vi "IR-sensor_labview_finalVersion.vi"() -> ()   [LabVIEW 2018]
uses:
  Downloads/Communicatie-met-Arduino-met-StateMachine-met-EventStructure (1).ctl
  <vilib>/Instr/_visa.llb/VISA Configure Serial Port (Instr).vi
panel:
  in  "VISA resource name":refnum<visa-resource-name>
  out "Absorberen":dbl(slide) scale=0.0..500.0
  in  "Clear Chart":bool
  out "Reflecteren":dbl(slide) scale=0.0..500.0
  out "Omgevings straling\nReferentie waarde":string
  in  "Kalibreren":bool
  out "Reflecteren":bool
  out "Absorberen":bool
  in  "Path":path
  out "Array":dbl[](array[numeric])
  in  "Wegschrijven":bool
  out "Status":T1
  in  "Baud rate":u32
  in  "Configure":bool
  in  "Stop":bool
  out "Waveform Chart":cluster{"decimal":u32, "Referentie":dbl}(graph)
  out "Huidige waarde":string
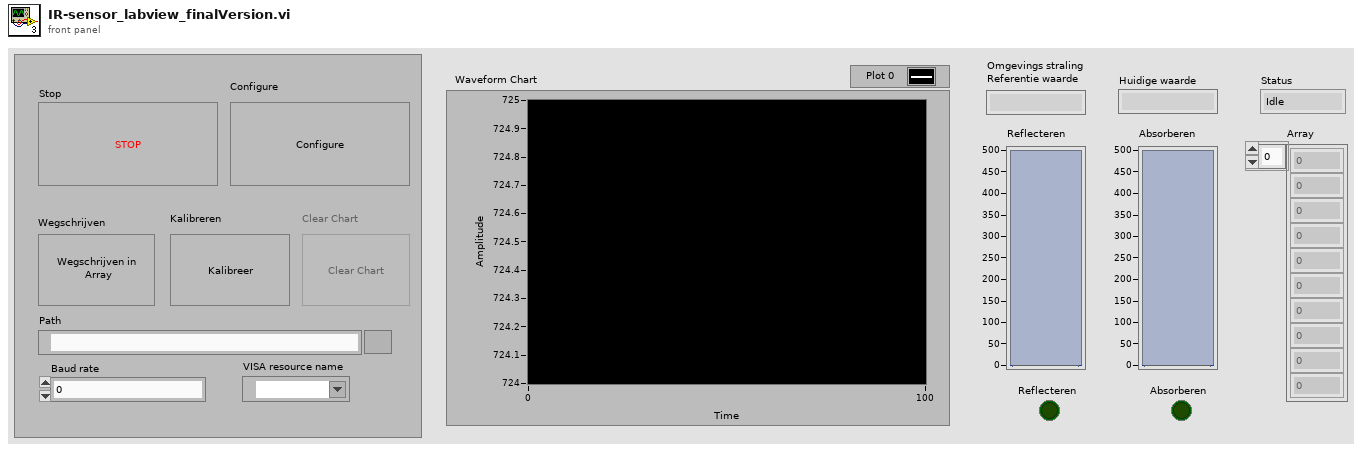
[diagram p1: front panel]
types:
  T1 = typedef "Communicatie-met-Arduino-met-StateMachine-met-EventStructure (1).ctl" = enum16{"Idle", "End", "Visualize", "Process", "Read", "Connect"}
  T2 = cluster{"COM Arduino":refnum<visa-resource-name>, "Baud rate 2":u32, "connect char":string, "buffer":string, "converted voltage":dbl, "decimal":u32, "value":i32, "saved values":dbl[], "refnum out":refnum<file>, "image":path, "ToArduino text":string, "Referentie":dbl}
  T3 = enum8{"Enabled", "Disabled", "Disabled and Grayed Out"}
  T4 = typedef "imagedata.ctl" = cluster{"image type":i32, "image depth":i32, "image":u8[], "mask":u8[], "colors":u32[], "Rectangle":cluster{"left":i16, "top":i16, "right":i16, "bottom":i16}}
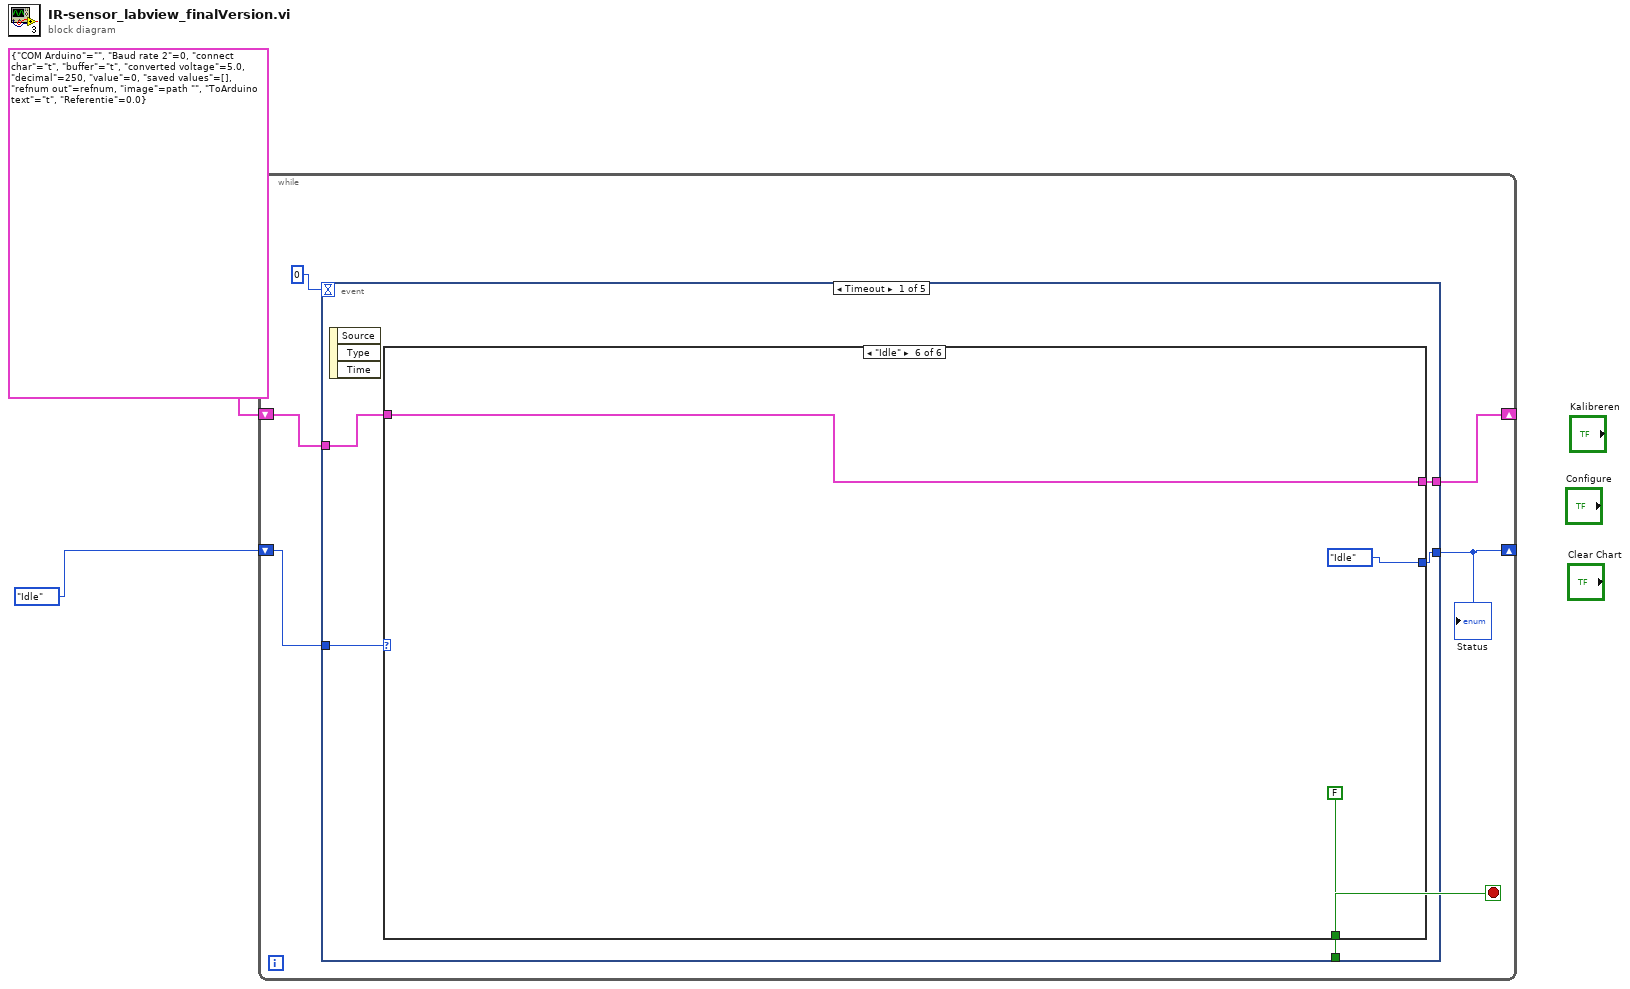
[diagram p0: block diagram]
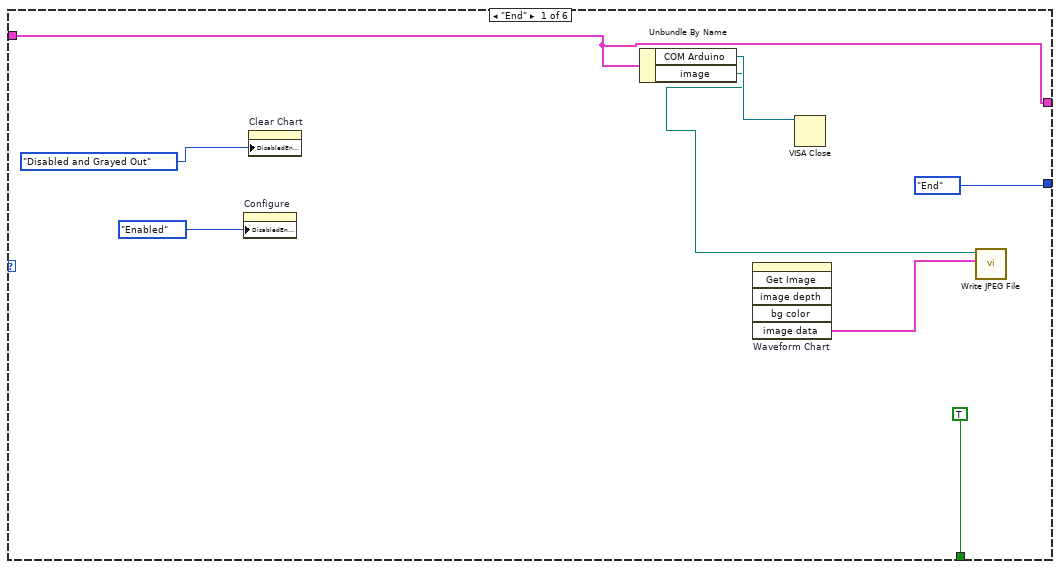
[diagram p2: hidden frame]
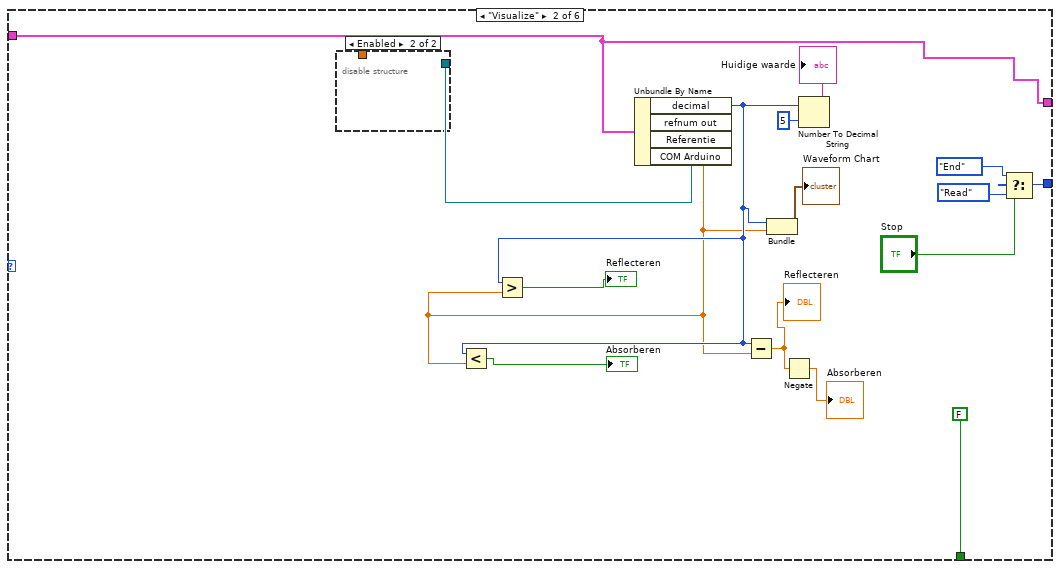
[diagram p3: hidden frame]
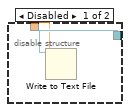
[diagram p4: hidden frame]
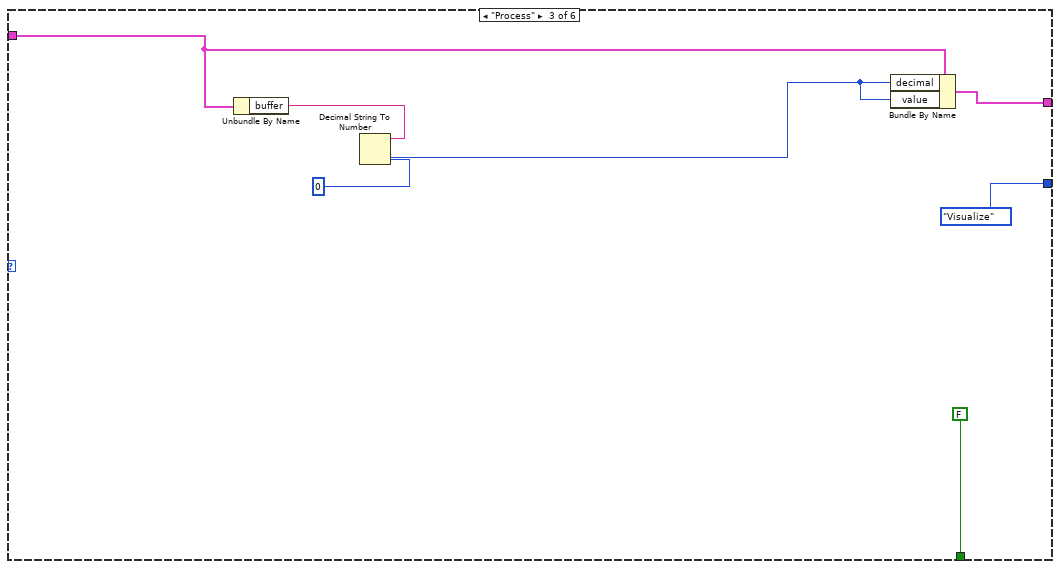
[diagram p5: hidden frame]
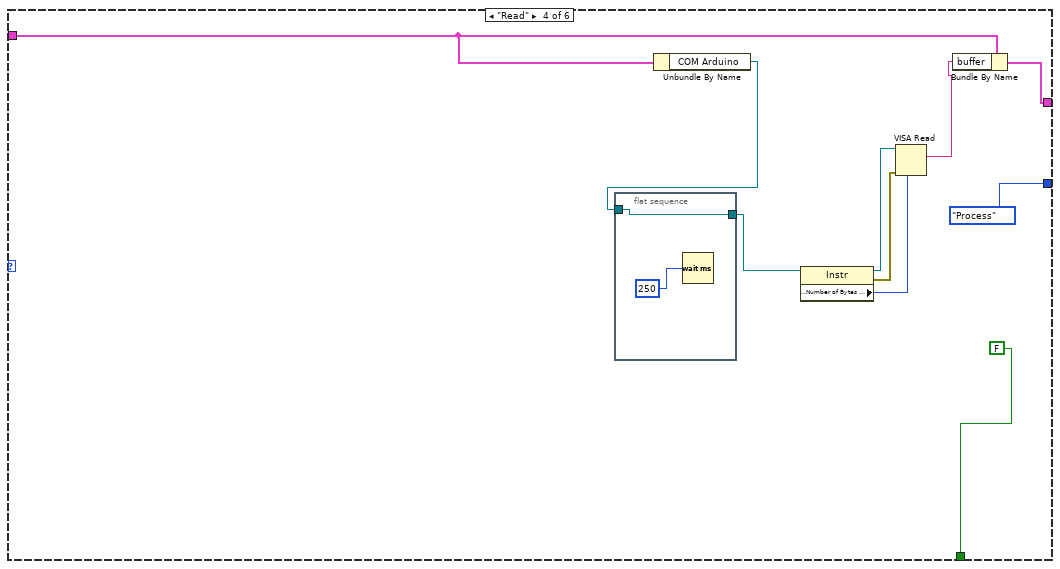
[diagram p6: hidden frame]
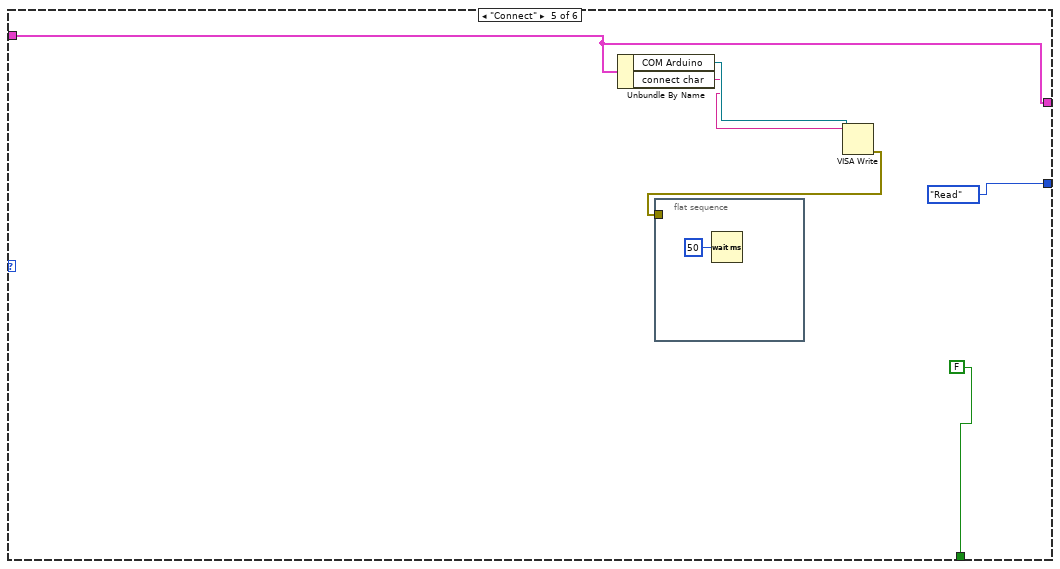
[diagram p7: hidden frame]
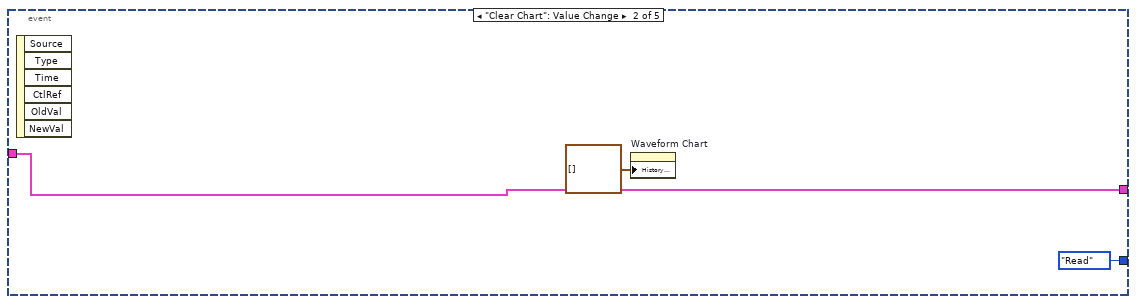
[diagram p8: hidden frame]
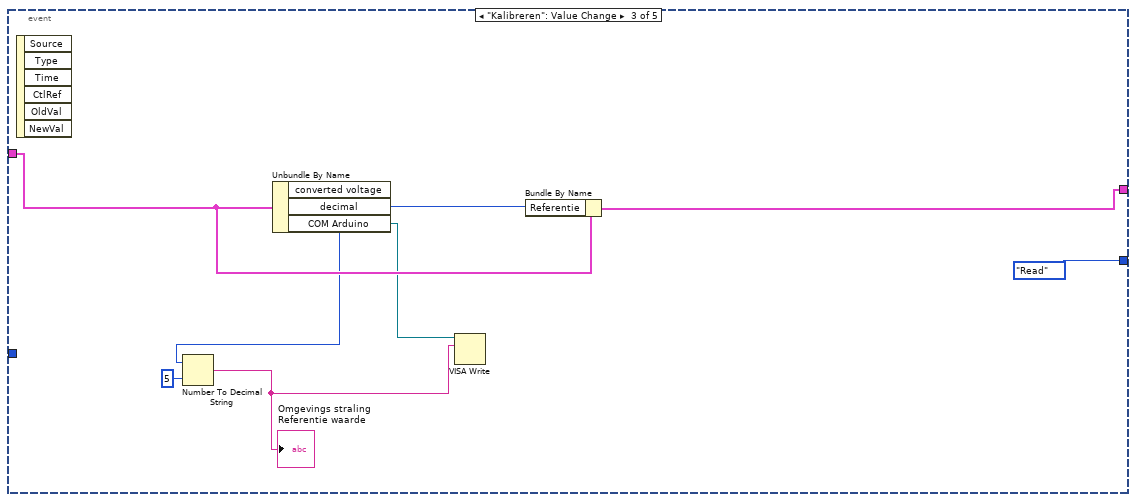
[diagram p9: hidden frame]
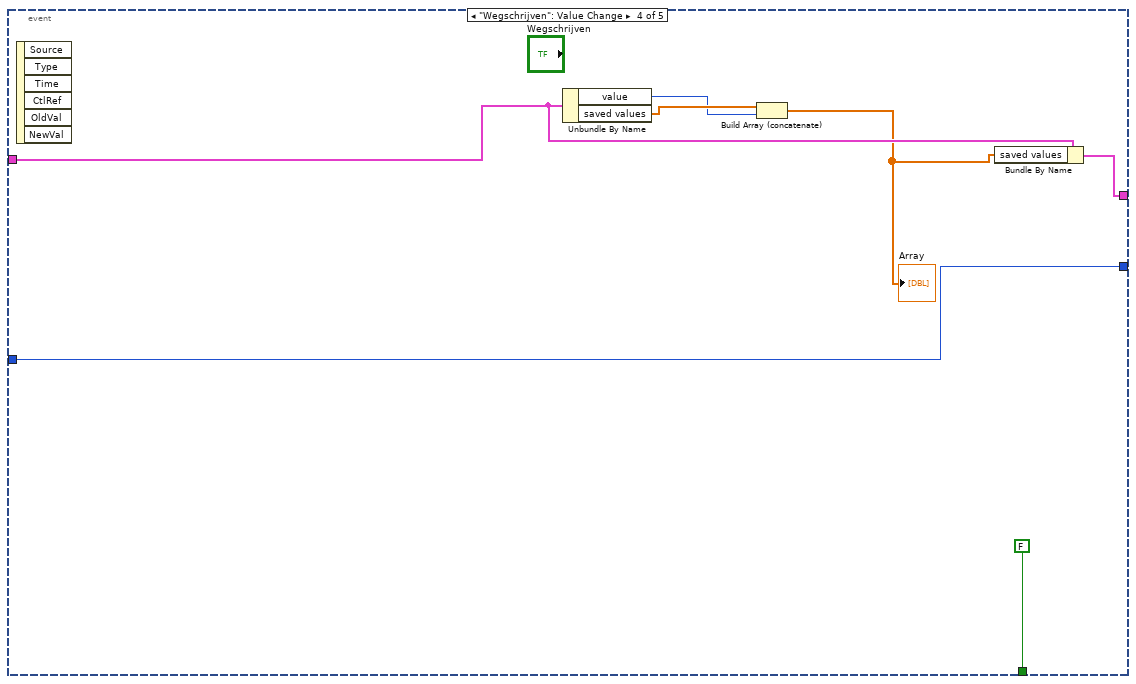
[diagram p10: hidden frame]
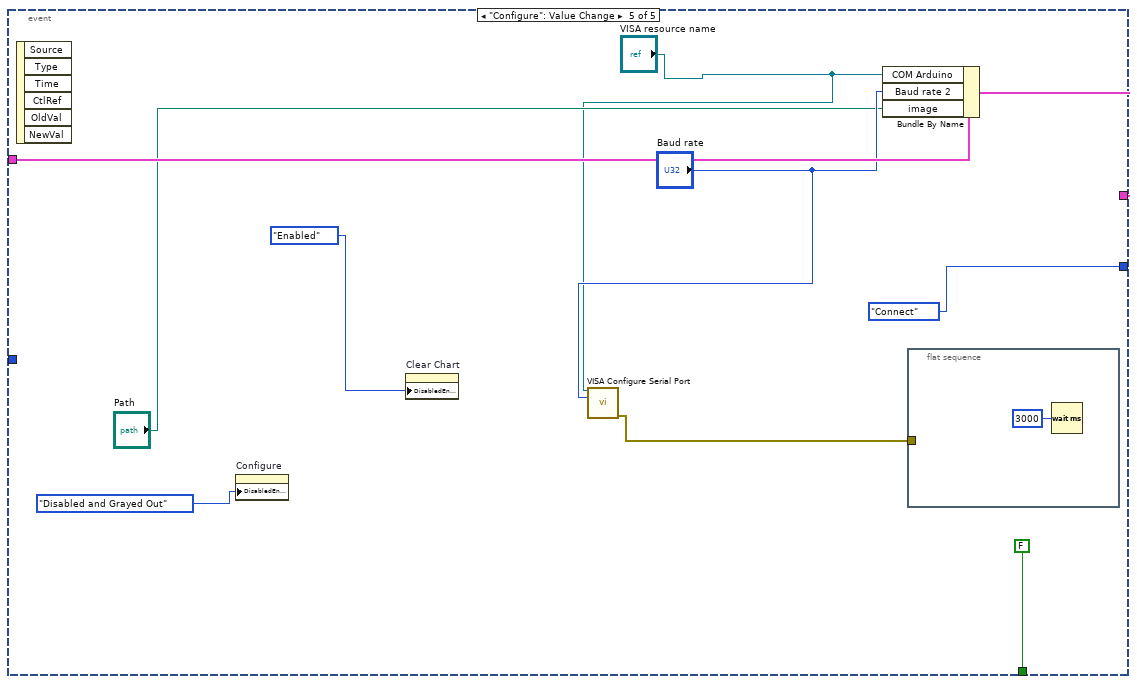
[diagram p11: hidden frame]
diagram:
  n1 = while {
    shift-right: [w5] -> _
    shift-left: Communicatie-met-Arduino-met-StateMachine-met-EventStructure_(1)."Idle" -> [w8]
    shift-right: [w6] -> _
    shift-left: T2 {"COM Arduino"="", "Baud rate 2"=0, "connect char"="t", "buffer"="t", "converted voltage"=5.0, "decimal"=250, "value"=0, "saved values"=[], "refnum out"=refnum, "image"=path "", "ToArduino text"="t", "Referentie"=0.0} ("Cluster") -> [w7]
    stop <- w4 stop-if-true
    n2 = event shown="[0] Timeout" {
      selector: _ -> [_ _ _ _ _]
      dyn-events: _ -> [_ _ _ _ _]
      timeout: 0 -> [_ _ _ _ _]
      tunnel: w8 -> [w13 _ _ w80 _]
      tunnel: w7 -> [w12 w70 w78 w83 w95]
      tunnel: [w11 w70 w77 w81 w94] -> w6
      tunnel: [w10 Communicatie-met-Arduino-met-StateMachine-met-EventStructure_(1)."Read" Communicatie-met-Arduino-met-StateMachine-met-EventStructure_(1)."Read" w80 Communicatie-met-Arduino-met-StateMachine-met-EventStructure_(1)."Connect"] -> w5
      tunnel: [w9 _ _ FALSE FALSE] -> w4
      event Timeout {
        n3 = event-data() -> ()  [unwired: 1 in, 3 out]
        n4 = case shown="\"Idle\"" w13 {
          tunnel: w12 -> [w18 w27 w45 w53 w62 w68]
          tunnel: [w18 w27 w44 w52 w62 w68] -> w11
          tunnel: [Communicatie-met-Arduino-met-StateMachine-met-EventStructure_(1)."End" w36 Communicatie-met-Arduino-met-StateMachine-met-EventStructure_(1)."Visualize" Communicatie-met-Arduino-met-StateMachine-met-EventStructure_(1)."Process" Communicatie-met-Arduino-met-StateMachine-met-EventStructure_(1)."Read" Communicatie-met-Arduino-met-StateMachine-met-EventStructure_(1)."Idle"] -> w10
          tunnel: [TRUE FALSE FALSE FALSE FALSE FALSE] -> w9
          frame "End" {
            n5 = property on="Configure" class="Bool"("DisabledEnum"=T3."Enabled" ("Disabled")) -> ()  [unwired: 2 in, 2 out]
            n6 = property on="Clear Chart" class="Bool"("DisabledEnum"=T3."Disabled and Grayed Out" ("Disabled")) -> ()  [unwired: 2 in, 2 out]
            n7 = Unbundle By Name(w18) -> ("COM Arduino"=w21:refnum<visa-resource-name>, "image"=w16:path)
            n8 = invoke on="Waveform Chart" class="WFChart (strict)" method="Get Image"() -> ("image data"=w17:T4)  [unwired: 6 in, 5 out]
            n9 = VISA Close(VISA resource name=w21) -> ()  [unwired: 1 in, 1 out]
            n10 = call <vilib>:"Write JPEG File.vi"("image data"=w17, "path to JPEG file"=w16) -> ()  [unwired: 8 in, 2 out]
          }
          frame "Visualize" {
            n11 = Unbundle By Name(w27) -> ("decimal"=w24:u32, "refnum out"=w33:refnum<file>, "Referentie"=w23:dbl)  [unwired: 1 out]
            n12 = disable-structure shown="Enabled" {
              disable-tunnel: w33 -> [w39 _]
              disable-tunnel: _ -> [w38 _]
              frame Disabled {
                n13 = Write to Text File(file (use dialog)=w39, text=w38) -> ()  [unwired: 2 in, 3 out]
              }
              frame Enabled {
              }
            }
            n14 = Less?(x=w24, y=w23) -> (x < y?=→"Absorberen":bool)
            n15 = Greater?(x=w24, y=w23) -> (0:→"Reflecteren":bool)
            n16 = Subtract(x=w24, y=w23) -> (x-y=w31:dbl)
            "Reflecteren" <- w31
            n17 = Bundle("decimal"=w24, "Referentie"=w23) -> (→"Waveform Chart":cluster{"decimal":u32, "Referentie":dbl})  [unwired: 1 in]
            n18 = Negate(x=w31) -> (-x=→"Absorberen":dbl)
            n19 = Number To Decimal String(number=w24, width (-)=i16 5) -> (decimal integer string=→"Huidige waarde":string)
            n20 = Select(t=Communicatie-met-Arduino-met-StateMachine-met-EventStructure_(1)."End", s="Stop", f=Communicatie-met-Arduino-met-StateMachine-met-EventStructure_(1)."Read") -> (s? t:f=w36:T1)
          }
          frame "Process" {
            n21 = Unbundle By Name(w45) -> ("buffer"=w46:string)
            n22 = Decimal String To Number(string=w46, default (0L)=0) -> (number=w40:i32)  [unwired: 1 in, 1 out]
            n23 = Bundle By Name(cluster=w45, "decimal"=w40, "value"=w40) -> (w44:T2)
          }
          frame "Read" {
            n24 = flat-sequence {
              tunnel: w49 -> [w57]
              tunnel: [w57] -> w48
              frame #0 {
                n25 = Wait (ms)(milliseconds to wait=u32 250 ("millisecond timer value")) -> ()  [unwired: 1 out]
              }
            }
            n26 = Unbundle By Name(w53) -> ("COM Arduino"=w49:refnum<visa-resource-name>)
            n27 = property class="Instr"(reference=w48) -> (reference out=w56:refnum<visa-resource-name>, error out=w54:errorcluster, "Serial Settings:Number of Bytes at Serial Port"=w55:u32)  [unwired: 1 in]
            n28 = VISA Read(VISA resource name=w56, byte count=w55, error in (no error)=w54) -> (read buffer=w47:string)  [unwired: 3 out]
            n29 = Bundle By Name(cluster=w53, "buffer"=w47) -> (w52:T2)
          }
          frame "Connect" {
            n30 = Unbundle By Name(w62) -> ("COM Arduino"=w64:refnum<visa-resource-name>, "connect char"=w63:string)
            n31 = flat-sequence {
              tunnel: w59 -> [_]
              frame #0 {
                n32 = Wait (ms)(milliseconds to wait=u32 50) -> ()  [unwired: 1 out]
              }
            }
            n33 = VISA Write(VISA resource name=w64, write buffer=w63) -> (error out=w59:errorcluster)  [unwired: 1 in, 2 out]
          }
          frame "Idle" {
          }
        }
      }
      event "Clear Chart": Value Change {
        n34 = event-data() -> ()  [unwired: 1 in, 6 out]
        n35 = property on="Waveform Chart" class="WFChart (strict)"("History Data"=cluster{"decimal":u32, "Referentie":dbl}[] []) -> ()  [unwired: 2 in, 2 out]
      }
      event "Kalibreren": Value Change {
        n36 = event-data() -> ()  [unwired: 1 in, 6 out]
        n37 = Unbundle By Name(w78) -> ("decimal"=w73:u32, "COM Arduino"=w74:refnum<visa-resource-name>)  [unwired: 1 out]
        n38 = Number To Decimal String(number=w73, width (-)=i16 5) -> (decimal integer string=w72:string)
        "Omgevings straling\nReferentie waarde" <- w72
        n39 = VISA Write(VISA resource name=w74, write buffer=w72) -> ()  [unwired: 1 in, 3 out]
        n40 = Bundle By Name(cluster=w78, "Referentie"=w73) -> (w77:T2)
      }
      event "Wegschrijven": Value Change {
        n41 = event-data() -> ()  [unwired: 1 in, 6 out]
        n42 = Unbundle By Name(w83) -> ("value"=w84:i32, "saved values"=w85:dbl[])
        n43 = Build Array (concatenate)(w85, w84) -> (w82:dbl[])
        "Array" <- w82
        n44 = Bundle By Name(cluster=w83, "saved values"=w82) -> (w81:T2)
      }
      event "Configure": Value Change {
        n45 = event-data() -> ()  [unwired: 1 in, 6 out]
        n46 = property on="Configure" class="Bool"("DisabledEnum"=T3."Disabled and Grayed Out" ("Disabled")) -> ()  [unwired: 2 in, 2 out]
        n47 = property on="Clear Chart" class="Bool"("DisabledEnum"=T3."Enabled" ("Disabled")) -> ()  [unwired: 2 in, 2 out]
        n48 = call-poly "VISA Configure Serial Port"("VISA resource name"="VISA resource name", "baud rate (9600)"="Baud rate") -> ("error out"=w92:errorcluster)  [unwired: 12 in, 1 out]
        n49 = Bundle By Name(cluster=w95, "COM Arduino"="VISA resource name", "Baud rate 2"="Baud rate", "image"="Path") -> (w94:T2)
        n50 = flat-sequence {
          tunnel: w92 -> [_]
          frame #0 {
            n51 = Wait (ms)(milliseconds to wait=u32 3000) -> ()  [unwired: 1 out]
          }
        }
      }
    }
    "Status" <- w5
  }
